vi "Periodic Check Distributed Manager Status.vi"(8 "error in (no error)":errorcluster, 11 "Error Manager in":refnum<class "Local Error Manager.lvclass">) -> (0 "error out":errorcluster, 3 "Error Manager out":refnum<class "Local Error Manager.lvclass">)   [LabVIEW 2026, in "TALOS.lvlib" / "Error Manager.lvlib" / "Local Error Manager.lvclass"]
uses:
  Local Error Manager.lvclass
  C:/LabVIEW Code/TALOS/talos/Father of all uServices/Father of all uServices/Father of all uServices.lvclass
  C:/LabVIEW Code/TALOS/talos/Internal uServices/System uServices/Error Manager/Error Manager.lvclass
  Father of all uServices/Father of all uServices/Father of all uServices.lvclass/Father of all uServices.ctl
  Ancestor/Ancestor/Ancestor.lvclass/Ancestor.ctl
  Error Manager.lvclass/Error Manager.ctl
  Read Distributed Error Manager Started flag.vi
  Read Distributed Mngr Status.vi
  Read Distributed flag.vi
  Write Distributed Error Manager Started flag.vi
  Write Distributed Mngr Status.vi
  Support VIs/Substitute Error.vi
  Support VIs/Generate Error.vi
  FGV/Error Memory/Get Error Description.vi
  Support VIs/Get PC name.vi
  Ancestor/Ancestor/Read ID.vi
  Support VIs/Get Class Name.vi
  <vilib>/Utility/error.llb/Clear Errors.vi
  FGV/Error Memory/Error Memory Core.vi
  <vilib>/AdvancedString/Delimited String to 1D String Array.vi
  <vilib>/AdvancedString/Delimited String to 1D String Array (string).vi
  Support VIs/Circus Root Path.vi
  FGV/Error Memory/Error Crt Lvl checker.vi
  FGV/Error Memory/Error Memory Core.vi/40c8088d-b597-4017-91af-faa98e00292e.vi
  FGV/Error Memory/Error Memory Core.vi/d4a3ab98-063c-4e44-b43d-fbdcfe6c2be2.vi
  Support VIs/Global Memory.vi
  <vilib>/Utility/LVClass/Get LV Class Name.vi
  Support VIs/Is in Packed Library.vi
  Support VIs/TALOS Root path.vi
  Support VIs/Read CSV worksheet.vi
  Support VIs/Global Constants.vi
  <vilib>/Utility/error.llb/General Error Handler.vi
  Support VIs/Error Log.vi
  Ancestor/Ancestor/Ancestor.lvclass
  <vilib>/Comparison/Equal/Equal Functor/Equal Functor.lvclass
  TALOS.lvlib
  Father of all uServices/Father of all uServices/Father of all uServices.lvclass
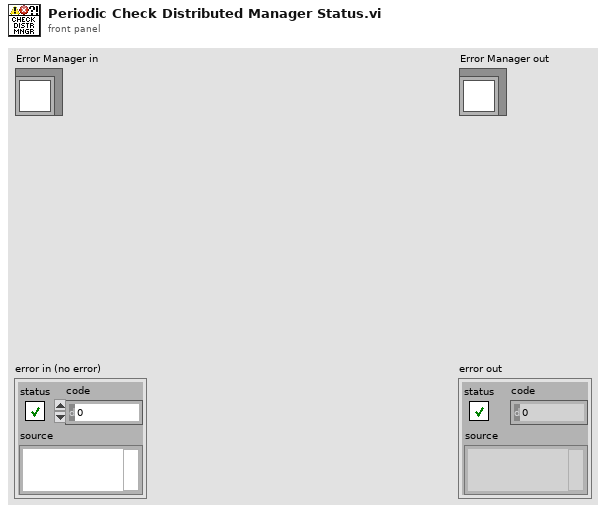
[diagram p1: front panel]
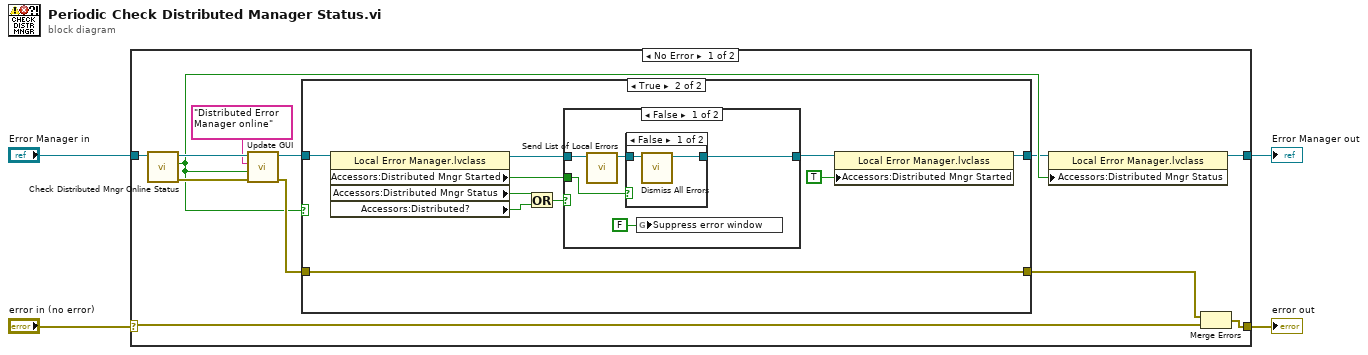
[diagram p0: block diagram]
diagram:
  n1 = case shown="No Error" "error in (no error)" {
    selector: "error in (no error)" -> [w16 w39]
    tunnel: [w14 w39] -> w3
    tunnel: [w5 w38] -> w1
    tunnel: "Error Manager in" -> [w13 w38]
    frame No Error {
      n2 = call "Check Distributed Mngr Online Status.vi"("Local Error Manager in"=w13) -> ("error out"=w9:errorcluster, "uService online"=w7:bool, "Local Error Manager out"=w12:refnum<class "Local Error Manager.lvclass">)  [unwired: 8 in]
      n3 = call "Update GUI.vi"("error in (no error)"=w9, "Data"=w7, "GUI Item Name"="Distributed Error Manager online", "uService Template in"=w12) -> ("error out"=w8:errorcluster, "uService Template out"=w11:refnum<class "Local Error Manager.lvclass">)  [unwired: 6 in]
      n4 = case shown="True" w7 {
        tunnel: w11 -> [w17 w28]
        tunnel: [w17 w20] -> w6
        tunnel: w8 -> [w18 w26]
        tunnel: [w18 w26] -> w15
        frame False {
        }
        frame True {
          n5 = property class="Local Error Manager.lvclass"(reference=w28) -> (reference out=w27:refnum<class "Local Error Manager.lvclass">, "Accessors:Distributed Mngr Started"=w22:bool, "Accessors:Distributed Mngr Status"=w23:bool, "Accessors:Distributed?"=w25:bool)  [unwired: 1 in, 1 out]
          n6 = Or(x=w23, y=w25) -> (x .or. y?=w24:bool)
          n7 = case shown="False" w24 {
            tunnel: w27 -> [w33 w37]
            tunnel: [w30 w37] -> w21
            tunnel: w22 -> [w29 _]
            frame False {
              n8 = call "Send List of Local Errors.vi"("Local Error Manager in"=w33) -> ("Local Error Manager out"=w31:refnum<class "Local Error Manager.lvclass">)  [unwired: 9 in, 1 out]
              n9 = case shown="False" w29 {
                tunnel: w31 -> [w35 w36]
                tunnel: [w34 w36] -> w30
                frame False {
                  n10 = call-dynamic "Dismiss All Errors.vi"("Error Manager in"=w35) -> ("Error Manager out"=w34:refnum<class "Local Error Manager.lvclass">)  [unwired: 9 in, 1 out]
                }
                frame True {
                }
              }
              n11 = global write "Global Memory.vi" "Suppress error window"(FALSE ("Suppress error window")) -> ()
            }
            frame True {
            }
          }
          n12 = property class="Local Error Manager.lvclass"(reference=w21, "Accessors:Distributed Mngr Started"=TRUE ("Distributed Mngr Started")) -> (reference out=w20:refnum<class "Local Error Manager.lvclass">)  [unwired: 1 in, 1 out]
        }
      }
      n13 = property class="Local Error Manager.lvclass"(reference=w6, "Accessors:Distributed Mngr Status"=w7) -> (reference out=w5:refnum<class "Local Error Manager.lvclass">)  [unwired: 1 in, 1 out]
      n14 = Merge Errors(w15, w16) -> (w14:errorcluster)
    }
    frame Error {
    }
  }
  "error out" <- w3
  "Error Manager out" <- w1
